vi "sub_Init_PSK_At_Rx.vi"(6 "Sync Bits":i32=20, 7 "synchronization parameters":T3={"expected sync location (symbols)"=-1, "sync sequence"=[], "sync location uncertainty (symbols)"=0, "sync indent (symbols)"=0} {"sync sequence" format="%.2f"}, 8 "error in (no error)":errorcluster, 9 "filter parameters":T4={"Alpha"=0.5, "Filter Length"=6, "TX Filter"=enum."Root Raised Cos"} {"Alpha" format="%.2f"}, 10 "PN sequence order (9)":i32=9, 11 "PSK Parameters":T2) -> (0 "error out":errorcluster, 3 "PSK Init Parameters":T1)   [LabVIEW 2023]
uses:
  <vilib>/addons/Modulation/Digital/General/MT Generate Bits (Galois, PN Order).vi
  <vilib>/addons/Modulation/Digital/Support/Common/Validators/mod_Generate Bits Validate.vi
  <vilib>/addons/Modulation/Analog/support/mod_Set Error Source.vi
  <vilib>/addons/Modulation/Digital/General/MT Generate PSK System Parameters(M).vi
  <vilib>/addons/Modulation/Digital/Support/Common/Validators/mod_Generate Filter Coefficients Validate.vi
  <vilib>/addons/Modulation/Digital/General/subVIs/mod_Generate Filter Coefficients.vi
  <vilib>/addons/Modulation/Digital/General/subVIs/mod_Generate Bits PN Sequence.vi
  <vilib>/addons/Modulation/Digital/General/MT Map Bits to PSK Symbols.vi
  <vilib>/addons/Modulation/niDMT.lvlib
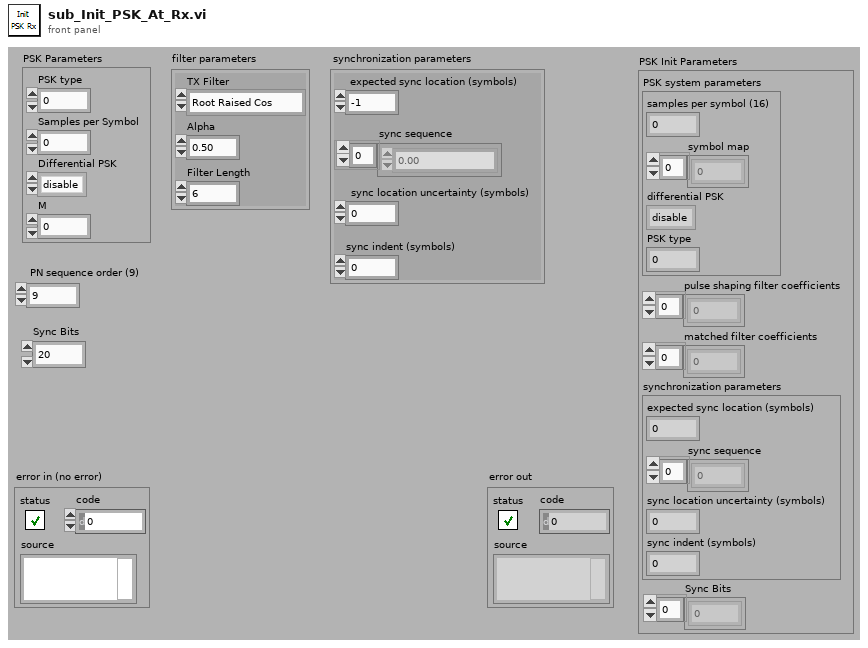
[diagram p1: front panel]
types:
  T1 = cluster{"PSK system parameters":cluster{"samples per symbol (16)":i32, "symbol map":cdb[], "differential PSK":enum16{"disable", "enable"}, "PSK type":u16}, "pulse shaping filter coefficients":dbl[], "matched filter coefficients":dbl[], "synchronization parameters":cluster{"expected sync location (symbols)":i32, "sync sequence":cdb[], "sync location uncertainty (symbols)":i32, "sync indent (symbols)":i32}, "Sync Bits":i8[]}
  T2 = cluster{"PSK type":u16, "Samples per Symbol":i32, "Differential PSK":enum16{"disable", "enable"}, "M":i32}
  T3 = cluster{"expected sync location (symbols)":i32, "sync sequence":cdb[], "sync location uncertainty (symbols)":i32, "sync indent (symbols)":i32}
  T4 = cluster{"Alpha":dbl, "Filter Length":i32, "TX Filter":enum16{"none", "Raised Cosine", "Root Raised Cos", "Gaussian"}}
  T5 = enum16{"FSK", "PSK", "QAM", "MSK", "PAM", "ASK", "CPM"}
  T6 = enum16{"none", "Raised Cosine", "Root Raised Cos", "Gaussian"}
  T7 = cluster{"samples per symbol (16)":i32, "symbol map":cdb[], "differential PSK":enum16{"disable", "enable"}, "PSK type":u16}
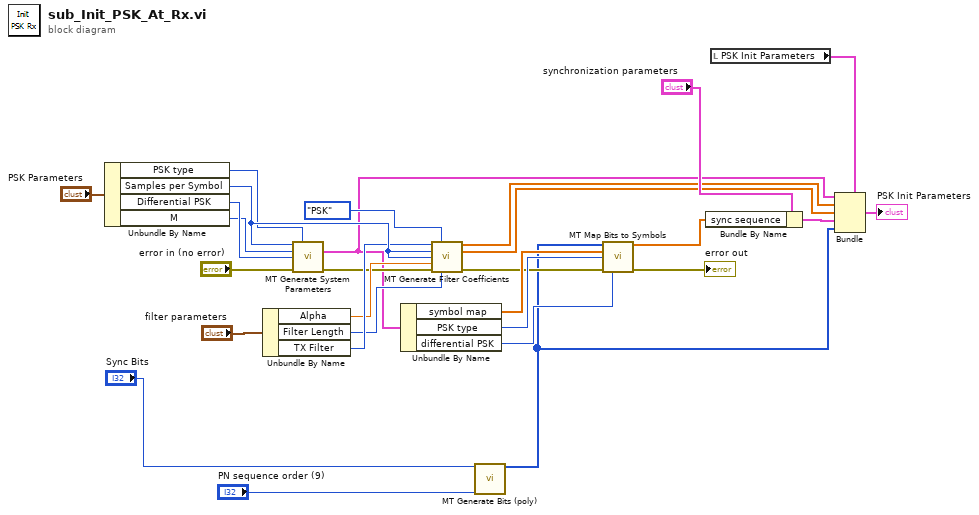
[diagram p0: block diagram]
diagram:
  n1 = Unbundle By Name("PSK Parameters") -> ("PSK type"=w25:u16, "Samples per Symbol"=w28:i32, "Differential PSK"=w27:enum16{"disable", "enable"}, "M"=w26:i32)
  n2 = Unbundle By Name("filter parameters") -> ("Alpha"=w16:dbl, "Filter Length"=w17:i32, "TX Filter"=w18:T6)
  n3 = call-poly <vilib>:"MT Generate System Parameters.vi"("samples per symbol (16)"=w28, "PSK type"=w25, "M-PSK (4)"=w26, "differential PSK"=w27, "error in (no error)"="error in (no error)") -> ("PSK system parameters"=w5:T7, "error out"=w14:errorcluster)  [unwired: 8 in, 1 out]
  n4 = Unbundle By Name(w5) -> ("symbol map"=w19:cdb[], "PSK type"=w20:u16, "differential PSK"=w21:enum16{"disable", "enable"})
  n5 = call <vilib>:"MT Generate Filter Coefficients.vi"("pulse shaping filter (none)"=w18, "modulation type"=T5."PSK", "pulse shaping samples per symbol (16)"=w28, "matched samples per symbol (16)"=w28, "filter parameter"=w16, "error in (no error)"=w14, "filter length (symbols)"=w17) -> ("pulse shaping filter coefficients"=w6:dbl[], "matched filter coefficients"=w11:dbl[], "error out"=w10:errorcluster)  [unwired: 6 in]
  n6 = call-poly <vilib>:"MT Generate Bits (poly).vi"("total bits (128)"="Sync Bits", "PN sequence order (9)"="PN sequence order (9)") -> ("output bit stream"=w3:i8[])  [unwired: 11 in, 2 out]
  n7 = call-poly <vilib>:"MT Map Bits to Symbols.vi"("input bit stream"=w3, "symbol map"=w19, "PSK type"=w20, "error in (no error)"=w10, "differential PSK"=w21) -> ("symbols"=w22:cdb[], "error out"=→"error out":errorcluster)  [unwired: 9 in]
  n8 = Bundle By Name(cluster="synchronization parameters", "sync sequence"=w22) -> (w12:T3)
  n9 = local read "PSK Init Parameters"() -> (w7:T1)
  n10 = Bundle(cluster=w7, "PSK system parameters"=w5, "pulse shaping filter coefficients"=w6, "matched filter coefficients"=w11, "synchronization parameters"=w12, "Sync Bits"=w3) -> (→"PSK Init Parameters":T1)
